vi "MotorError.vi"(9 "args":string[](array[string]), 10 "motorErrorType":T1) -> (0 "error out":errorcluster)   [LabVIEW 2016, in "Stepper Motor Controller.lvlib" / "KST101.lvclass"]
uses:
  KST101.lvclass
  KST-MotorError.ctl
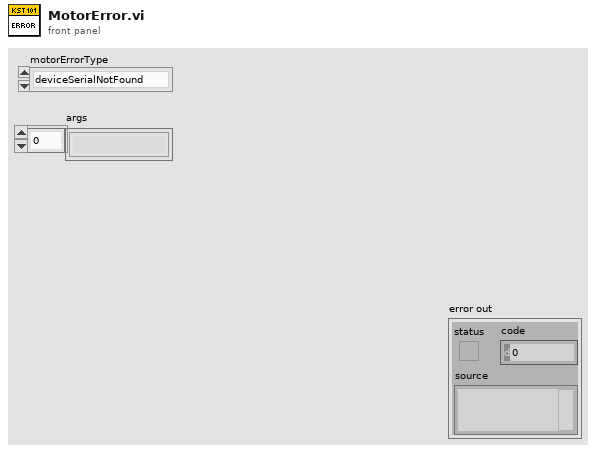
[diagram p1: front panel]
types:
  T1 = typedef "Stepper Motor Controller.lvlib/KST101.lvclass/KST-MotorError.ctl" = enum16{"deviceSerialNotFound"}
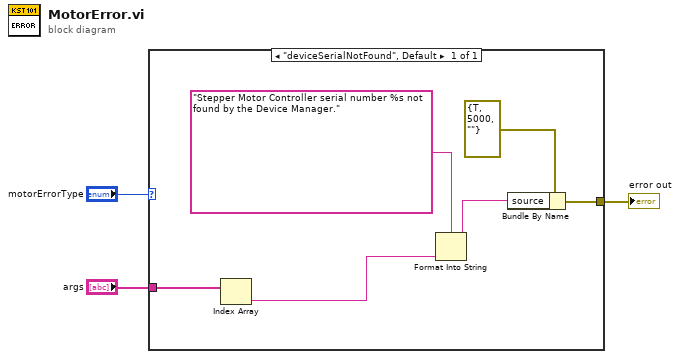
[diagram p0: block diagram]
diagram:
  n1 = case shown="\"deviceSerialNotFound\", Default" "motorErrorType" {
    tunnel: [w8] -> w1
    tunnel: "args" -> [w5]
    frame "deviceSerialNotFound", Default {
      n2 = Index Array(array=w5) -> (element=w4:string)  [unwired: 1 in]
      n3 = Format Into String(format string="Stepper Motor Controller serial number %s not found by the Device Manager." ("source"), w4) -> (resulting string=w6:string)  [unwired: 2 in, 1 out]
      n4 = Bundle By Name(cluster=errorcluster {"status"=TRUE, "code"=5000, "source"=""} ("error out"), "source"=w6) -> (w8:errorcluster)
    }
  }
  "error out" <- w1
